vi "BMS_Extended_Data_view.vi"() -> ()   [LabVIEW 2018]
uses:
  Type_Def/TypeDef_BMSDatas.ctl
  Type_Def/TypeDef_BMSStatuss.ctl
  <vilib>/Platform/TimedLoop/XDataNode/timing_clust.ctl
  <vilib>/Platform/TimedLoop/XDataNode/nitl_modes.ctl
  <vilib>/Platform/TimedLoop/XDataNode/wakeup.ctl
  Type_Def/Master_DataControl.ctl
  Type_Def/TypeDef_cRIODatas.ctl
  Type_Def/Type_Def IMUDatas.ctl
  Type_Def/TypeDef FixedMotorData.ctl
  <vilib>/Platform/TimedLoop/XDataNode/XDataNode.xnode
  <vilib>/Platform/TimedLoop/XDataNode/XDNodeRunTimeDep.lvlib
panel:
  in  "stop":bool
  out "BMS Data":T1
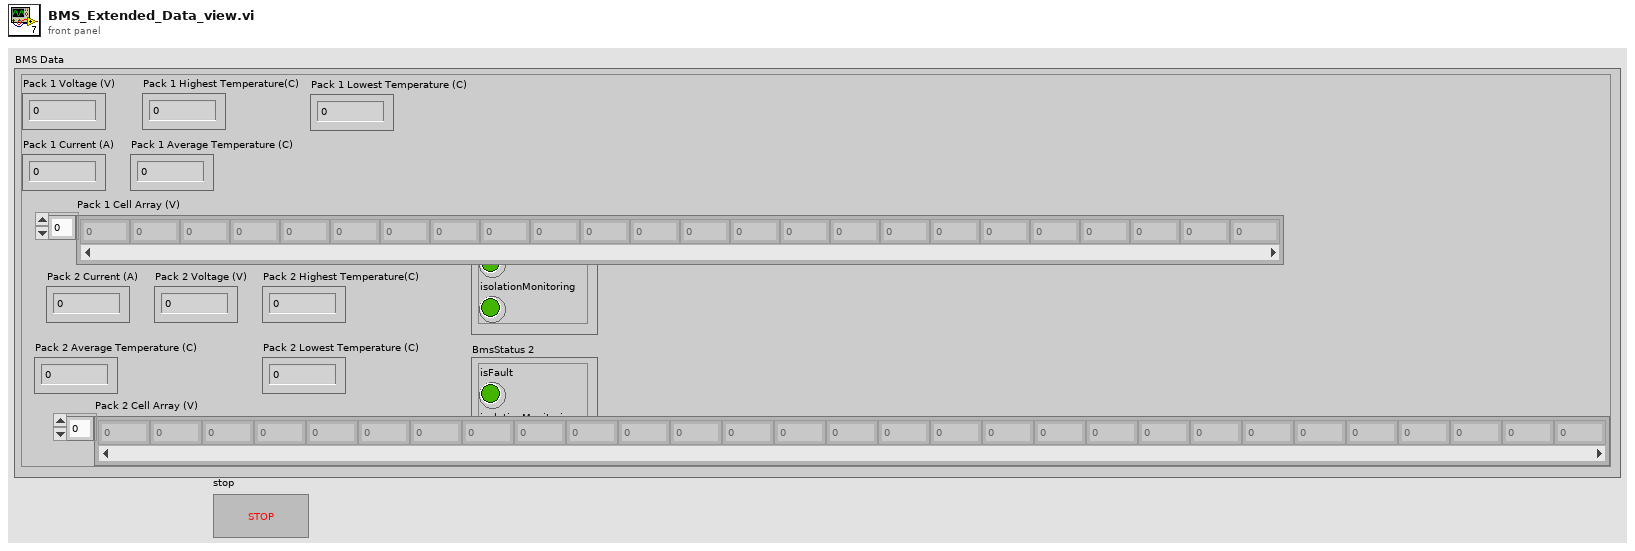
[diagram p1: front panel]
types:
  T1 = typedef "TypeDef_BMSDatas.ctl" = cluster{"Pack 1 Current (A)":dbl, "Pack 1 Voltage (V)":dbl, "Pack 1 Highest Temperature(C)":dbl, "BmsStatus1":T2, "Pack 2 Current (A)":dbl, "Pack 2 Voltage (V) ":dbl, "Pack 2 Highest Temperature(C) ":dbl, "BmsStatus 2":T2, "Pack 1 Cell Array (V)":dbl[], "Pack 2 Cell Array (V)":dbl[], "Pack 1 Lowest Temperature (C)":dbl, "Pack 1 Average Temperature (C)":dbl, "Pack 2 Average Temperature (C)":dbl, "Pack 2 Lowest Temperature (C)":dbl}
  T2 = typedef "TypeDef_BMSStatuss.ctl" = cluster{"isFault":bool, "isolationMonitoring":bool}
  T3 = typedef "XDNodeRunTimeDep.lvlib/timing_clust.ctl" = cluster{"Expected End [f-1]":u64, "Actual End [f-1]":u64, "Finished Late? [f-1]":bool, "Expected End [i-1]":u64, "Actual End [i-1]":u64, "Finished Late? [i-1]":bool, "Expected Start [i]":u64, "Actual Start [i]":u64, "Expected Start [f]":u64, "Actual Start [f]":u64, "Source Name":string, "Structure Name":string, "Period":i64, "Deadline":i64, "Offset":i64, "Start":i64, "Priority":i32, "Timeout":i32, "Mode":T4, "Wakeup Reason":T5, "Error":errorcluster, "Source Type":string, "Secondary Source Type":string, "Global End Time":u64, "Global Start Time":u64, "Frame Duration":u64, "Iteration Duration":u64, "Assigned CPU":i32, "I/O Scan Engine Mode":u32}
  T4 = typedef "XDNodeRunTimeDep.lvlib/nitl_modes.ctl" = enum32{"No Change", "Process missed periods, maintain original phase", "Discard missed periods, maintain original phase", "Process missed periods, ignore original phase", "Discard missed periods, ignore original phase"}
  T5 = typedef "XDNodeRunTimeDep.lvlib/wakeup.ctl" = enum32{"Normal", "Aborted", "Asynchronous wakeup", "Timing source error", "Timed loop error", "Timeout"}
  T6 = typedef "Master_DataControl.ctl" = cluster{"cRIO Data":T7, "IMU Data":T8, "BMS Data":T1, "Motor Data":T9}
  T7 = typedef "TypeDef_cRIODatas.ctl" = cluster{"HallEffect Right (cm)":dbl, "HallEffect Left (cm)":dbl, "Optical Sensor 1 (V)":dbl, "Optical Sensor 2 (V)":dbl, "24V Voltage  (V)":dbl, "24V Current (A)":dbl, "Contactor H1 Continuity":dbl, "Contactor L1 Continuity ":dbl, "Contactor H2 Continuity":dbl, "Contactor L2 Continuity ":dbl, "Brake PT(psig)":dbl, "Pump PT (psig)":dbl, "24V Temp   (C)":dbl, "Tank PT(psig) ":dbl, "ABS Pressure 1 (psig)":dbl, "ABS Pressure 2 (psig) ":dbl, "Displacement (ft)":dbl, "Velocity (ft/s)":dbl, "Time (ms)":dbl, "PV 1 Temp (C)":dbl, "PV2 Temp (C)":dbl}
  T8 = typedef "Type_Def IMUDatas.ctl" = cluster{"y acceleration (g)":dbl, "Pressure (psia)":dbl, "Temperature (C)":dbl}
  T9 = typedef "TypeDef FixedMotorData.ctl" = cluster{" Velocity (RPM)":dbl, " MotorTemp(C)":dbl, " ControlTemp(C)":dbl, " DcLinkVolt(V)":dbl, " ErrorCode":dbl, "IsAlive":bool, "motorStatus":cluster{"isReady":bool, "isOn":bool, "isOperEn":bool, "isFault":bool, "isVoltEn":bool, "targetReached":bool, "isWarning":bool}, "motorControllerState":u16}
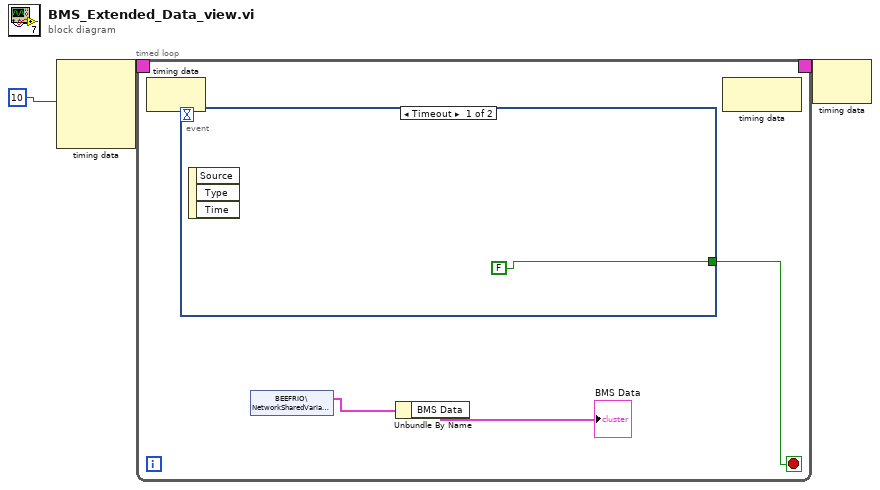
[diagram p0: block diagram]
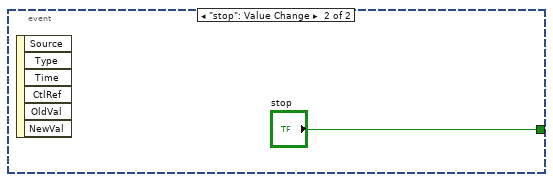
[diagram p2: hidden frame]
diagram:
  n1 = node-c288(10) -> (w3:T3)  [unwired: 3 in]
  n2 = timed-loop {
    timing: w3 -> [_]
    timing-out: [_] -> w2
    stop <- w4 stop-if-true
    n3 = node-c288() -> ()  [unwired: 1 in, 1 out]
    n4 = event shown="[0] Timeout" {
      selector: _ -> [_ _]
      dyn-events: _ -> [_ _]
      timeout: _ -> [_ _]
      tunnel: [FALSE "stop"] -> w4
      event Timeout {
        n5 = event-data() -> ()  [unwired: 1 in, 3 out]
      }
      event "stop": Value Change {
        n6 = event-data() -> ()  [unwired: 1 in, 6 out]
      }
    }
    n7 = shared-variable "BEEFRIO\\NetworkSharedVariable.lvlib\\AllData"() -> (w6:T6)  [unwired: 1 in, 1 out]
    n8 = Unbundle By Name(w6) -> ("BMS Data"=→"BMS Data":T1)
    n9 = node-c288() -> ()  [unwired: 1 in, 1 out]
  }
  n10 = node-c288(w2) -> ()  [unwired: 1 out]
